vi "Write_ERD_Data_to_File.vi"(0 "refnum in":refnum<file>, 7 "ERD_Data_Bundled_In":T1, 11 "Error In":errorcluster) -> (4 "refnum out":refnum<file>, 15 "Error Out":errorcluster)   [LabVIEW 2014]
uses:
  type defs/ERD_Data_Bundled.ctl
  type defs/ATC_Data.ctl
  type defs/Redundant.ctl
  type defs/Version.ctl
  type defs/Algorithms.ctl
  type defs/ERD_Always_Show.ctl
  type defs/Fault_Table_Info.ctl
  type defs/Cycle_Diag.ctl
panel:
  # "Wet Load Size"
  # "Dry Load Size"
  # "OOB"
  # "Software Version"
  # "Critical Version"
  # "Non-Critical"
  # "XML Crit Ver"
  # "XML Non-Crit"
  # "Daily Build"
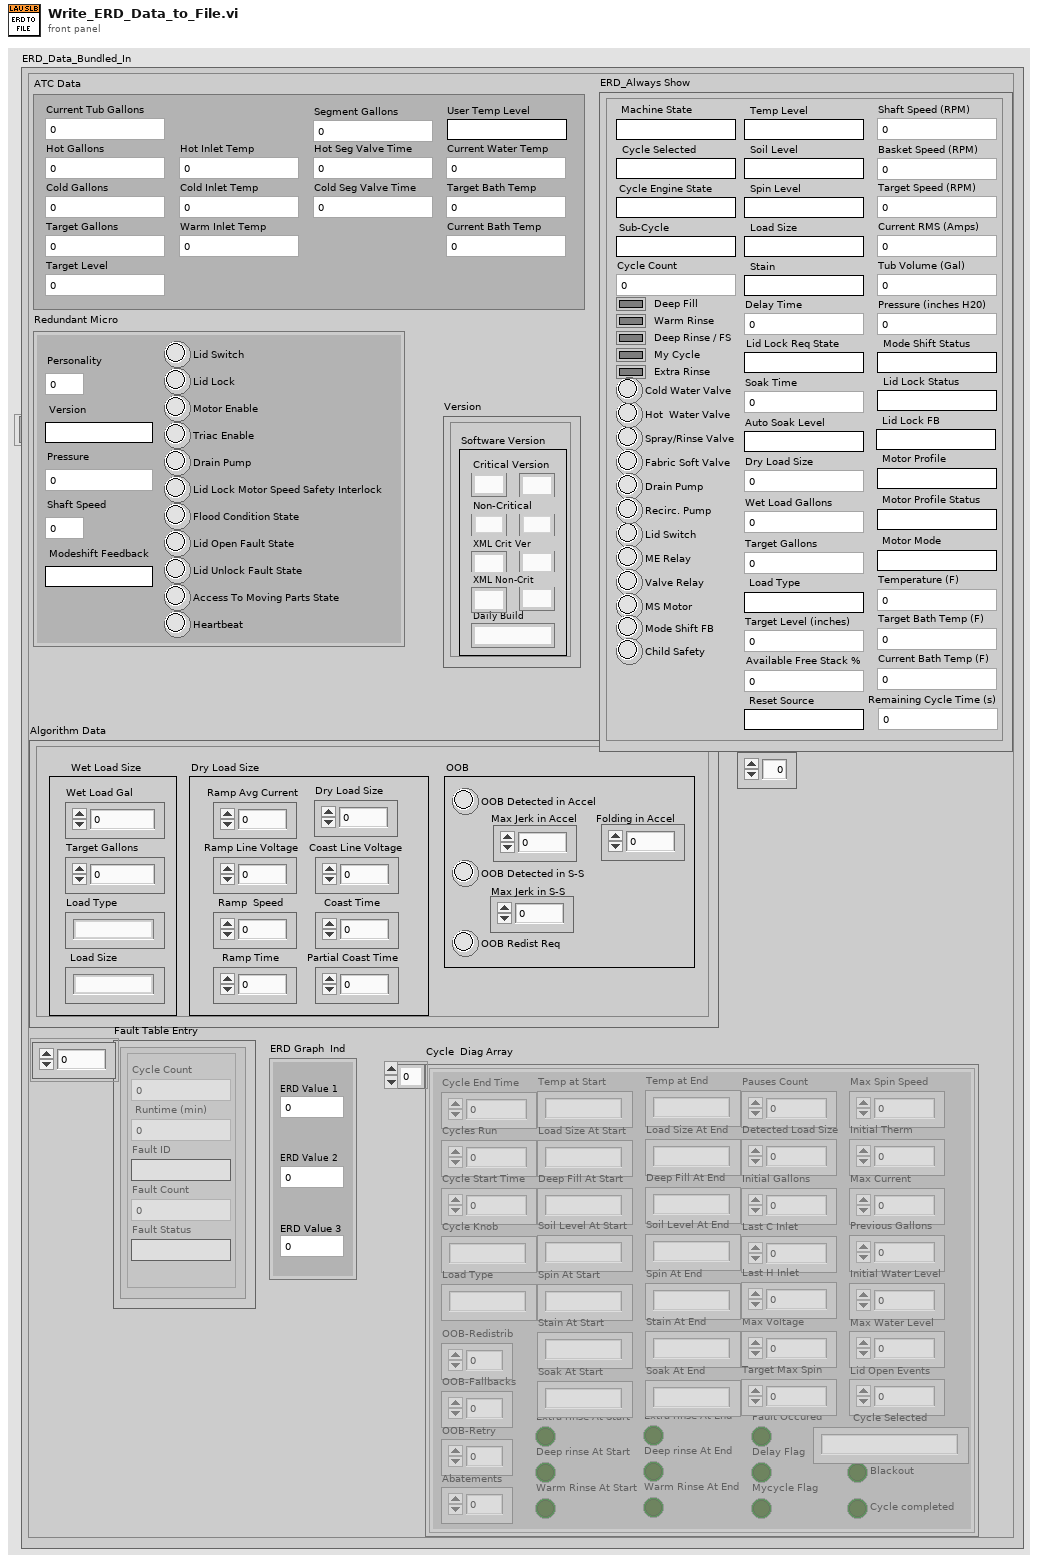
[diagram p1: front panel]
types:
  T1 = typedef "ERD_Data_Bundled.ctl" = cluster{"ATC Data":T2, "Redundant Micro":T3, "Version":T4, "Algorithm Data":T5, "ERD_Always Show":T6, "ERD Graph  Ind":cluster{"ERD Value 1":dbl, "ERD Value 2":dbl, "ERD Value 3":dbl}, "Personality Set":u8, "Fault Table Entry":T7[], "Cycle  Diag Array":T8[]}
  T2 = typedef "ATC_Data.ctl" = cluster{"Current Tub Gallons":dbl, "Hot Gallons":dbl, "Cold Gallons":dbl, "Target Gallons":dbl, "Current Water Temp":dbl, "Target Level":u32, "Target Bath Temp":dbl, "Current Bath Temp ":dbl, "Cold Inlet Temp":dbl, "Hot Inlet Temp":dbl, "Warm Inlet Temp":dbl, "Hot Seg Valve Time":u16, "Cold Seg Valve Time ":u16, "User Temp Level":string, "Segment Gallons":dbl}
  T3 = typedef "Redundant.ctl" = cluster{"Version":string, "Personality":u8, "Pressure ":dbl, "Shaft Speed":u16, "Modeshift Feedback":string, "Lid Switch":bool, "Lid Lock":bool, "Triac Enable":bool, "Drain Pump":bool, "Lid Lock Motor Speed Safety Interlock":bool, "Flood Condition State":bool, "Lid Open Fault State":bool, "Access To Moving Parts State":bool, "Heartbeat":bool, "Motor Enable":bool, "Lid Unlock Fault State":bool}
  T4 = typedef "Version.ctl" = cluster{"Critical Major":string, "Critical Minor":string, "Non-Critical Minor":string, "Non-Critical Major":string, "XML Crit Minor":string, "XMLCrit Major":string, "Daily Rev":string, "XML Non-crit Minor":string, "Xml Non-crit Major":string}
  T5 = typedef "Algorithms.ctl" = cluster{"Wet Load Gal":dbl, "Target Gallons":dbl, "Load Type":string, "Load Size":string, "Coast Time":u16, "Ramp Time":u16, "Ramp  Speed":u16, "Ramp Avg Current":dbl, "OOB Redist Req":bool, "OOB Detected in S-S":bool, "Folding in Accel":i32, "Max Jerk in Accel":i32, "Max Jerk in S-S":i32, "OOB Detected in Accel":bool, "Partial Coast Time":u16, "Dry Load Size":dbl, "Ramp Line Voltage ":dbl, "Coast Line Voltage":dbl}
  T6 = typedef "ERD_Always_Show.ctl" = cluster{"Basket Speed (RPM)":u16, "Machine State":string, "Tub Volume (Gal)":dbl, "Pressure (inches H20)":dbl, "Lid Switch ":bool, "Current RMS (Amps)":dbl, "Cycle Selected":string, "Lid Lock Status":string, "Mode Shift Status":string, "Spray/Rinse Valve":bool, "Fabric Soft Valve":bool, "Drain Pump":bool, "Recirc. Pump":bool, "Cycle Engine State":string, "Hot  Water Valve":bool, "Cold Water Valve":bool, "Motor Profile":string, "Motor Profile Status":string, "Motor Mode":string, "ME Relay":bool, "Cycle Count":u32, "Deep Rinse / FS":bool, "My Cycle":bool, "Soil Level":string, "Spin Level":string, "Stain":string, "Temp Level":string, "Load Size":string, "Delay Time":u16, "Soak Time":u16, "Deep Fill":bool, "Warm Rinse":bool, "Auto Soak Level":string, "Extra Rinse":bool, "Wet Load Gallons":dbl, "Target Gallons":dbl, "Sub-Cycle":string, "Load Type":string, "Target Level (inches)":u32, "Valve Relay":bool, "Dry Load Size":dbl, "Shaft Speed (RPM) ":u16, "MS Motor":bool, "Mode Shift FB":bool, "Target Bath Temp (F)":dbl, "Temperature (F)":dbl, "Current Bath Temp (F)":dbl, "Lid Lock FB":string, "Lid Lock Req State":string, "Remaining Cycle Time (s)":u32, "Available Free Stack %":u8, "Child Safety":bool, "Target Speed (RPM)":u16, "Reset Source":string}
  T7 = typedef "Fault_Table_Info.ctl" = cluster{"Cycle Count":u32, " Runtime (min) ":u32, "Fault Status":string, "Fault ID":string, "Fault Count":u16}
  T8 = typedef "Cycle_Diag.ctl" = cluster{"Cycle End Time":u32, "Cycles Run":u32, "Cycle Start Time":u32, "Cycle Knob":string, "Load Type":string, "OOB-Redistrib":u8, "OOB-Fallbacks":u8, "OOB-Retry":u8, "Temp at Start":string, "Load Size At Start":string, "Deep Fill At Start":string, "Soil Level At Start":string, "Spin At Start":string, "Extra rinse At Start":bool, "Deep rinse At Start":bool, "Stain At Start":string, "Soak At Start":string, "Warm Rinse At Start":bool, "Temp at End":string, "Load Size At End":string, "Deep Fill At End":string, "Soil Level At End":string, "Spin At End":string, "Extra rinse At End":bool, "Deep rinse At End":bool, "Stain At End":string, "Soak At End":string, "Warm Rinse At End":bool, "Pauses Count":u8, "Fault Occured":bool, "Delay Flag":bool, "Mycycle Flag":bool, "Blackout":bool, "Cycle completed":bool, "Detected Load Size":dbl, "Initial Gallons":dbl, "Last C Inlet ":dbl, "Max Voltage":dbl, "Target Max Spin":u16, "Max Spin Speed":u16, "Initial Therm":dbl, "Max Current":dbl, "Previous Gallons":dbl, "Initial Water Level":dbl, "Max Water Level":dbl, "Abatements ":u8, "Lid Open Events":u8, "Cycle Selected":string, "Last H Inlet ":dbl}
  T9 = cluster{"ERD Value 1":dbl, "ERD Value 2":dbl, "ERD Value 3":dbl}
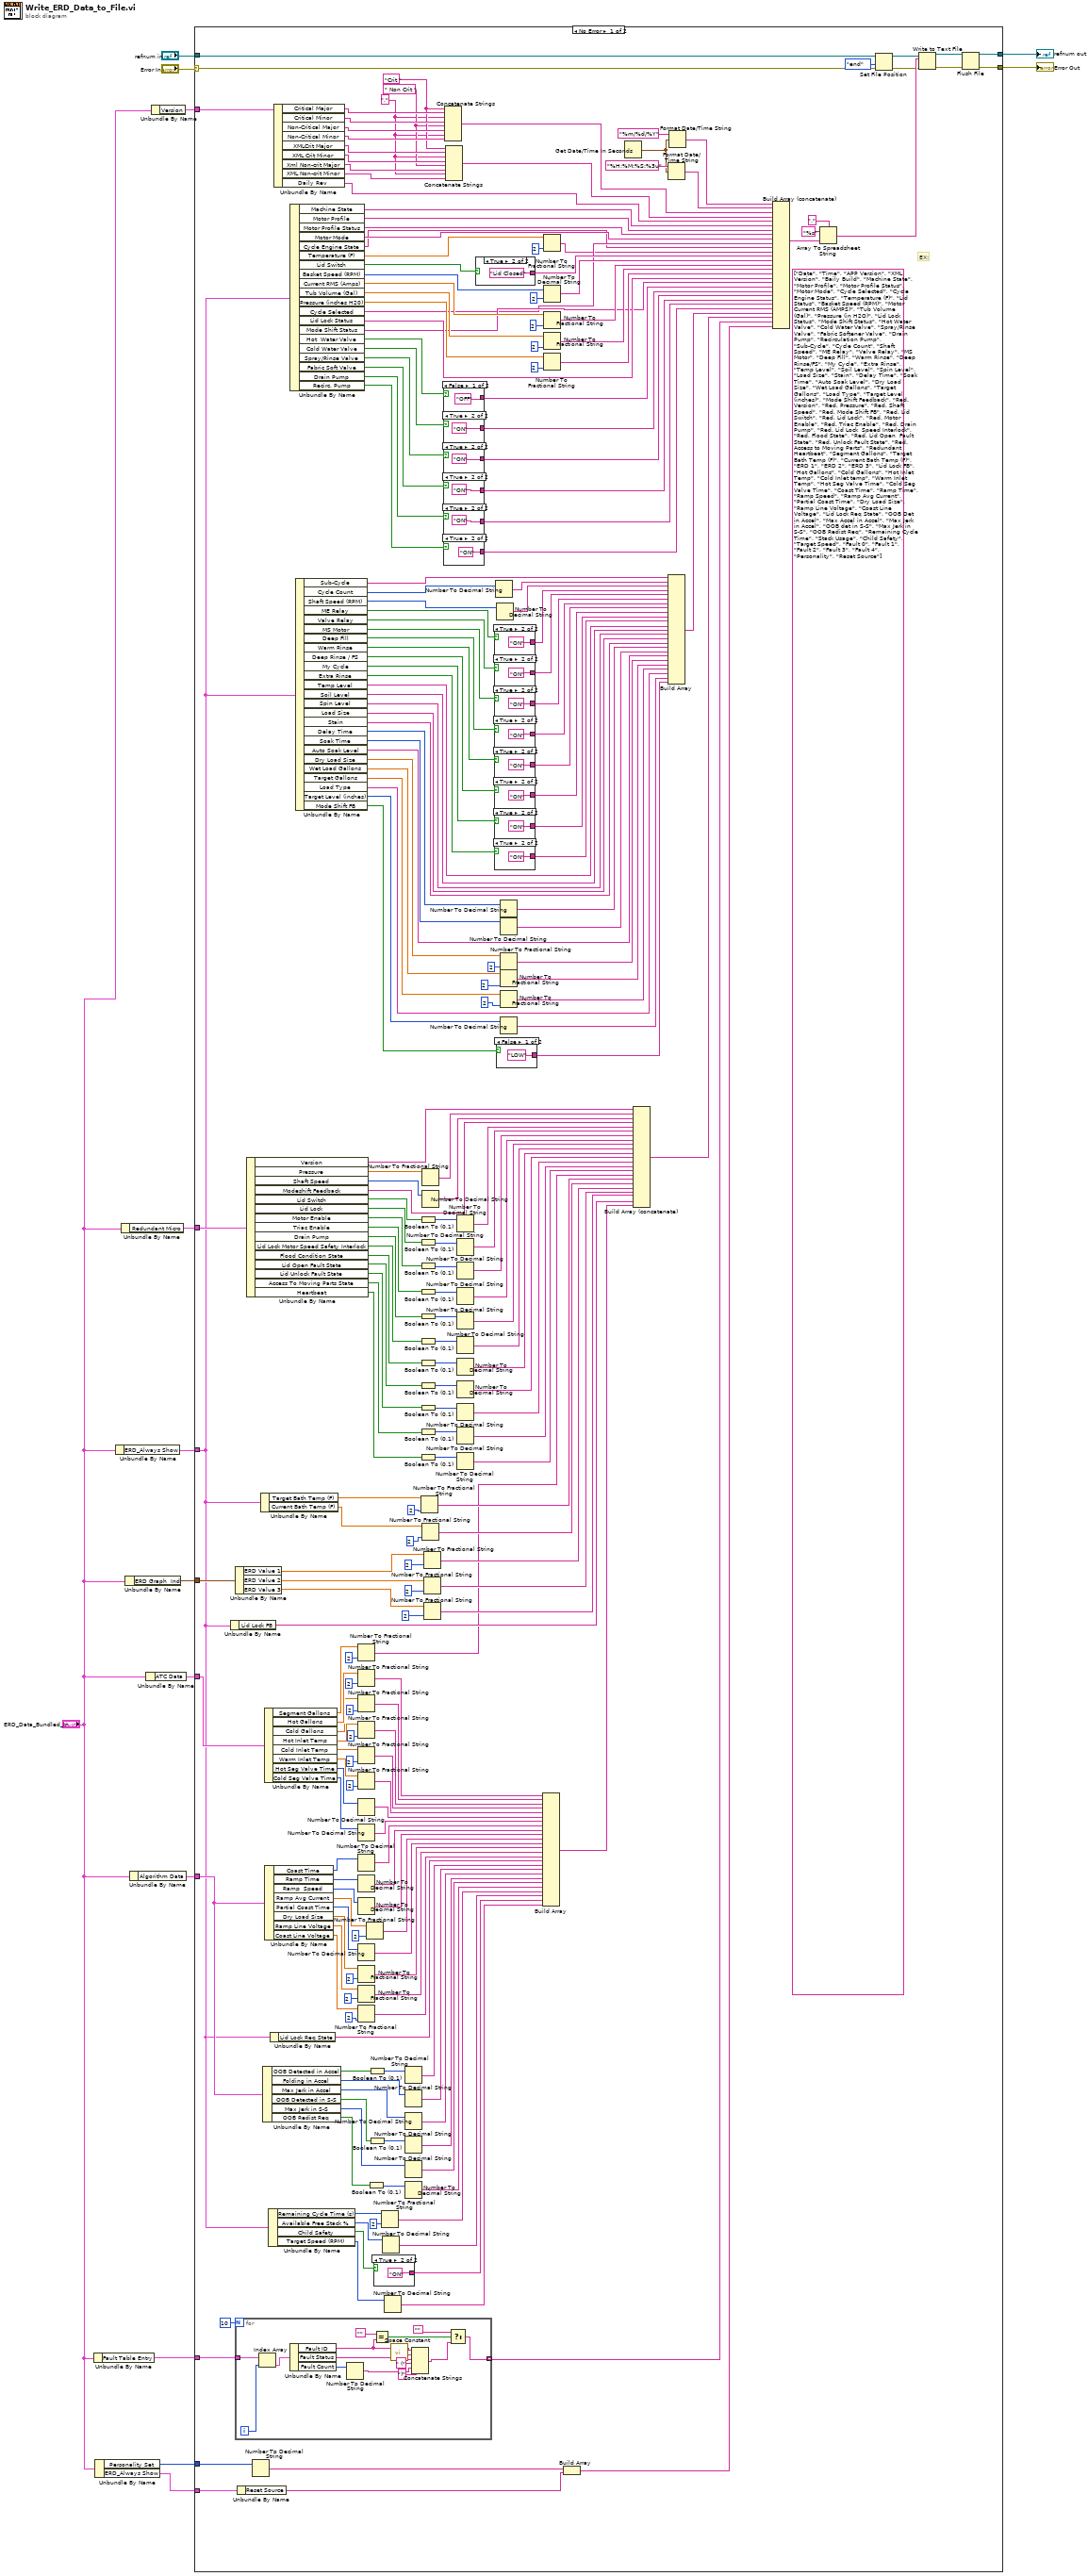
[diagram p0: block diagram]
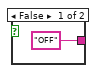
[diagram p2: hidden frame]
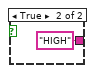
[diagram p3: hidden frame]
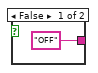
[diagram p4: hidden frame]
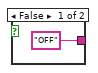
[diagram p5: hidden frame]
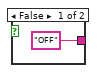
[diagram p6: hidden frame]
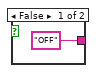
[diagram p7: hidden frame]
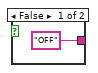
[diagram p8: hidden frame]
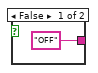
[diagram p9: hidden frame]
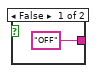
[diagram p10: hidden frame]
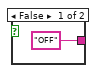
[diagram p11: hidden frame]
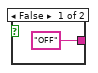
[diagram p12: hidden frame]
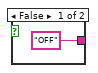
[diagram p13: hidden frame]
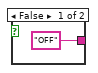
[diagram p14: hidden frame]
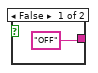
[diagram p15: hidden frame]
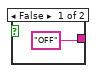
[diagram p16: hidden frame]
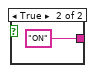
[diagram p17: hidden frame]
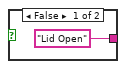
[diagram p18: hidden frame]
diagram:
  n1 = Unbundle By Name("ERD_Data_Bundled_In") -> ("Fault Table Entry"=w1:T7[])
  n2 = Unbundle By Name("ERD_Data_Bundled_In") -> ("Personality Set"=w3:u8, "ERD_Always Show"=w2:T6)
  n3 = Unbundle By Name("ERD_Data_Bundled_In") -> ("ERD_Always Show"=w7:T6)
  n4 = Unbundle By Name("ERD_Data_Bundled_In") -> ("Redundant Micro"=w8:T3)
  n5 = Unbundle By Name("ERD_Data_Bundled_In") -> ("ERD Graph  Ind"=w5:T9)
  n6 = Unbundle By Name("ERD_Data_Bundled_In") -> ("Algorithm Data"=w9:T5)
  n7 = Unbundle By Name("ERD_Data_Bundled_In") -> ("ATC Data"=w10:T2)
  n8 = Unbundle By Name("ERD_Data_Bundled_In") -> ("Version"=w6:T4)
  n9 = case shown="No Error" "Error In" {
    selector: "Error In" -> [w232 w318]
    tunnel: [w24 w317] -> w13
    tunnel: "refnum in" -> [w235 w317]
    tunnel: [w23 w318] -> w11
    tunnel: w6 -> [w174 _]
    tunnel: w8 -> [w157 _]
    tunnel: w5 -> [w112 _]
    tunnel: w10 -> [w104 _]
    tunnel: w9 -> [w71 _]
    tunnel: w7 -> [w22 _]
    tunnel: w3 -> [w21 _]
    tunnel: w2 -> [w20 _]
    tunnel: w1 -> [w16 _]
    frame No Error {
      (unwired) string[] ["Date", "Time", "APP Version", "XML Version", "Baily Build", "Machine State", "Motor Profile", "Motor Profile Status", "Motor Mode", "Cycle Selected", "Cycle Engine Status", "Temperature (F)", "Lid Status", "Basket Speed (RPM)", "Motor Current RMS (AMPS)", "Tub Volume (Gal)", "Pressure (in H2O)", "Lid Lock Status", "Mode Shift Status", "Hot Water Valve", "Cold Water Valve", "Spray/Rinse Valve", "Fabric Softener Valve", "Drain Pump", "Recirculation Pump", "Sub-Cycle", "Cycle Count", "Shaft Speed", "ME Relay", "Valve Relay", "MS Motor", "Deep Fill", "Warm Rinse", "Deep Rinse/FS", "My Cycle", "Extra Rinse", "Temp Level", "Soil Level", "Spin Level", "Load Size", "Stain", "Delay Time", "Soak Time", "Auto Soak Level", "Dry Load Size", "Wet Load Gallons", "Target Gallons", "Load Type", "Target Level (inches)", "Mode Shift Feedback", "Red. Version", "Red. Pressure", "Red. Shaft Speed", "Red. Mode Shift FB", "Red. Lid Switch", "Red. Lid Lock", "Red. Motor Enable", "Red. Triac Enable", "Red. Drain Pump", "Red. Lid Lock  Speed Interlock", "Red. Flood State", "Red. Lid Open  Fault State", "Red. Unlock Fault State", "Red. Access to Moving Parts", "Redundant Heartbeat", "Segment Gallons", "Target Bath Temp (F)", "Current Bath Temp (F)", "ERD 1", "ERD 2", "ERD 3", "Lid Lock FB", "Hot Gallons", "Cold Gallons", "Hot Inlet Temp", "Cold Inlet temp", "Warm Inlet Temp", "Hot Seg Valve Time", "Cold Seg Valve Time", "Coast Time", "Ramp Time", "Ramp Speed", "Ramp Avg Current", "Partial Coast Time", "Dry Load Size", "Ramp Line Voltage", "Coast Line Voltage", "Lid Lock Req State", "OOB Det in Accel", "Max Accel in Accel", "Max Jerk in Accel", "OOB det in S-S", "Max Jerk in S-S", "OOB Redist Req", "Remaining Cycle Time", "Stack Usage", "Child Safety", "Target Speed", "Fault 0", "Fault 1", "Fault 2", "Fault 3", "Fault 4", "Personality", "Reset Source"]
      w166 = " Non Crit " ("element")
      w164 = "." ("element")
      w169 = "Crit " ("element")
      # "EX:"
      n10 = Unbundle By Name(w22) -> ("Lid Lock FB"=w105:string)
      n11 = Unbundle By Name(w112) -> ("ERD Value 1"=w111:dbl, "ERD Value 2"=w110:dbl, "ERD Value 3"=w109:dbl)
      n12 = for {
        N: 10 -> [_]
        tunnel: [w272] -> w27 mode=indexing
        tunnel: w16 -> [w270]
        i -> [w268]
        n13 = Index Array(array=w270, index=w268) -> (element=w269:T7)
        n14 = Unbundle By Name(w269) -> ("Fault ID"=w275:string, "Fault Status"=w280:string, "Fault Count"=w282:u16)
        n15 = Number To Decimal String(number=w282) -> (decimal integer string=w278:string)  [unwired: 1 in]
        n16 = Equal?(x="", y=w275) -> (x = y?=w274:bool)
        n17 = call <vilib>:"Space Constant.vi"() -> ("String"=w281:string)
        n18 = Concatenate Strings(w275, w281, w280, " (" ("string"), w278, ")" ("string")) -> (w273:string)
        n19 = Select(t="", s=w274, f=w273) -> (s? t:f=w272:string)
      }
      n20 = Unbundle By Name(w20) -> ("Reset Source"=w18:string)
      n21 = Unbundle By Name(w157) -> ("Version"=w156:string, "Pressure"=w155:dbl, "Shaft Speed"=w153:u16, "Modeshift Feedback"=w151:string, "Lid Switch"=w148:bool, "Lid Lock"=w138:bool, "Motor Enable"=w137:bool, "Triac Enable"=w136:bool, "Drain Pump"=w135:bool, "Lid Lock Motor Speed Safety Interlock"=w134:bool, "Flood Condition State"=w133:bool, "Lid Open Fault State"=w132:bool, "Lid Unlock Fault State"=w130:bool, "Access To Moving Parts State"=w129:bool, "Heartbeat"=w128:bool)
      n22 = Number To Decimal String(number=w21) -> (decimal integer string=w19:string)  [unwired: 1 in]
      n23 = Unbundle By Name(w22) -> ("Target Bath Temp (F)"=w116:dbl, "Current Bath Temp (F)"=w114:dbl)
      n24 = Unbundle By Name(w71) -> ("OOB Detected in Accel"=w69:bool, "Folding in Accel"=w67:i32, "Max Jerk in Accel"=w65:i32, "OOB Detected in S-S"=w63:bool, "Max Jerk in S-S"=w62:i32, "OOB Redist Req"=w60:bool)
      n25 = Unbundle By Name(w104) -> ("Segment Gallons"=w38:dbl, "Hot Gallons"=w103:dbl, "Cold Gallons"=w102:dbl, "Hot Inlet Temp"=w101:dbl, "Cold Inlet Temp"=w100:dbl, "Warm Inlet Temp"=w99:dbl, "Hot Seg Valve Time"=w98:u16, "Cold Seg Valve Time"=w97:u16)
      n26 = Unbundle By Name(w71) -> ("Coast Time"=w88:u16, "Ramp Time"=w87:u16, "Ramp  Speed"=w86:u16, "Ramp Avg Current"=w85:dbl, "Partial Coast Time"=w84:u16, "Dry Load Size"=w83:dbl, "Ramp Line Voltage"=w82:dbl, "Coast Line Voltage"=w81:dbl)
      n27 = Unbundle By Name(w22) -> ("Remaining Cycle Time (s)"=w35:u32, "Available Free Stack %"=w33:u8, "Child Safety"=w31:bool, "Target Speed (RPM)"=w29:u16)
      n28 = Unbundle By Name(w22) -> ("Lid Lock Req State"=w72:string)
      n29 = Unbundle By Name(w174) -> ("Critical Major"=w173:string, "Critical Minor"=w172:string, "Non-Critical Major"=w171:string, "Non-Critical Minor"=w170:string, "XMLCrit Major"=w168:string, "XML Crit Minor"=w167:string, "Xml Non-crit Major"=w165:string, "XML Non-crit Minor"=w163:string, "Daily Rev"=w158:string)
      n30 = Unbundle By Name(w22) -> ("Machine State"=w266:string, "Motor Profile"=w265:string, "Motor Profile Status"=w226:string, "Motor Mode"=w224:string, "Cycle Engine State"=w220:string, "Temperature (F)"=w225:dbl, "Lid Switch"=w257:bool, "Basket Speed (RPM)"=w258:u16, "Current RMS (Amps)"=w250:dbl, "Tub Volume (Gal)"=w261:dbl, "Pressure (inches H20)"=w260:dbl, "Cycle Selected"=w221:string, "Lid Lock Status"=w249:string, "Mode Shift Status"=w248:string, "Hot  Water Valve"=w247:bool, "Cold Water Valve"=w246:bool, "Spray/Rinse Valve"=w245:bool, "Fabric Soft Valve"=w244:bool, "Drain Pump"=w239:bool, "Recirc. Pump"=w238:bool)
      n31 = Unbundle By Name(w22) -> ("Sub-Cycle"=w218:string, "Cycle Count"=w217:u32, "Shaft Speed (RPM)"=w215:u16, "ME Relay"=w213:bool, "Valve Relay"=w212:bool, "MS Motor"=w211:bool, "Deep Fill"=w210:bool, "Warm Rinse"=w209:bool, "Deep Rinse / FS"=w208:bool, "My Cycle"=w207:bool, "Extra Rinse"=w206:bool, "Temp Level"=w198:string, "Soil Level"=w197:string, "Spin Level"=w196:string, "Load Size"=w195:string, "Stain"=w194:string, "Delay Time"=w193:u16, "Soak Time"=w192:u16, "Auto Soak Level"=w191:string, "Dry Load Size"=w190:dbl, "Wet Load Gallons"=w189:dbl, "Target Gallons"=w188:dbl, "Load Type"=w182:string, "Target Level (inches)"=w180:u32, "Mode Shift FB"=w178:bool)
      n32 = Number To Fractional String(number=w38, precision (6)=i16 2) -> (F-format string=w37:string)  [unwired: 2 in]
      n33 = Number To Fractional String(number=w103, precision (6)=i16 2) -> (F-format string=w96:string)  [unwired: 2 in]
      n34 = Number To Fractional String(number=w102, precision (6)=i16 2) -> (F-format string=w95:string)  [unwired: 2 in]
      n35 = Number To Fractional String(number=w101, precision (6)=i16 2) -> (F-format string=w94:string)  [unwired: 2 in]
      n36 = Number To Fractional String(number=w100, precision (6)=i16 2) -> (F-format string=w93:string)  [unwired: 2 in]
      n37 = Number To Fractional String(number=w99, precision (6)=i16 2) -> (F-format string=w92:string)  [unwired: 2 in]
      n38 = Number To Decimal String(number=w98) -> (decimal integer string=w91:string)  [unwired: 1 in]
      n39 = Number To Decimal String(number=w97) -> (decimal integer string=w90:string)  [unwired: 1 in]
      n40 = Number To Decimal String(number=w88) -> (decimal integer string=w80:string)  [unwired: 1 in]
      n41 = Number To Decimal String(number=w87) -> (decimal integer string=w79:string)  [unwired: 1 in]
      n42 = Number To Decimal String(number=w86) -> (decimal integer string=w78:string)  [unwired: 1 in]
      n43 = Number To Decimal String(number=w84) -> (decimal integer string=w76:string)  [unwired: 1 in]
      n44 = Number To Fractional String(number=w83, precision (6)=i16 2) -> (F-format string=w75:string)  [unwired: 2 in]
      n45 = Number To Fractional String(number=w82, precision (6)=i16 2) -> (F-format string=w74:string)  [unwired: 2 in]
      n46 = Number To Fractional String(number=w81, precision (6)=i16 2) -> (F-format string=w73:string)  [unwired: 2 in]
      n47 = Number To Fractional String(number=w85, precision (6)=i16 2) -> (F-format string=w77:string)  [unwired: 2 in]
      n48 = Boolean To (0,1)(Boolean=w60) -> (0, 1=w61:i16)
      n49 = Boolean To (0,1)(Boolean=w69) -> (0, 1=w70:i16)
      n50 = Boolean To (0,1)(Boolean=w63) -> (0, 1=w64:i16)
      n51 = case shown="True" w31 {
        tunnel: ["OFF" "ON"] -> w30
        frame False {
        }
        frame True {
        }
      }
      n52 = Number To Fractional String(number=w35, precision (6)=i16 2) -> (F-format string=w34:string)  [unwired: 2 in]
      n53 = Number To Decimal String(number=w33) -> (decimal integer string=w32:string)  [unwired: 1 in]
      n54 = Number To Decimal String(number=w29) -> (decimal integer string=w28:string)  [unwired: 1 in]
      n55 = Number To Decimal String(number=w70) -> (decimal integer string=w68:string)  [unwired: 1 in]
      n56 = Number To Decimal String(number=w67) -> (decimal integer string=w66:string)  [unwired: 1 in]
      n57 = Number To Decimal String(number=w65) -> (decimal integer string=w59:string)  [unwired: 1 in]
      n58 = Number To Decimal String(number=w64) -> (decimal integer string=w58:string)  [unwired: 1 in]
      n59 = Number To Decimal String(number=w62) -> (decimal integer string=w57:string)  [unwired: 1 in]
      n60 = Number To Decimal String(number=w61) -> (decimal integer string=w56:string)  [unwired: 1 in]
      n61 = Boolean To (0,1)(Boolean=w148) -> (0, 1=w150:i16)
      n62 = Boolean To (0,1)(Boolean=w138) -> (0, 1=w147:i16)
      n63 = Boolean To (0,1)(Boolean=w137) -> (0, 1=w146:i16)
      n64 = Boolean To (0,1)(Boolean=w136) -> (0, 1=w145:i16)
      n65 = Boolean To (0,1)(Boolean=w135) -> (0, 1=w144:i16)
      n66 = Boolean To (0,1)(Boolean=w134) -> (0, 1=w143:i16)
      n67 = Boolean To (0,1)(Boolean=w133) -> (0, 1=w142:i16)
      n68 = Boolean To (0,1)(Boolean=w132) -> (0, 1=w141:i16)
      n69 = Boolean To (0,1)(Boolean=w130) -> (0, 1=w140:i16)
      n70 = Boolean To (0,1)(Boolean=w129) -> (0, 1=w139:i16)
      n71 = Boolean To (0,1)(Boolean=w128) -> (0, 1=w131:i16)
      n72 = Number To Fractional String(number=w116, precision (6)=i16 2) -> (F-format string=w115:string)  [unwired: 2 in]
      n73 = Number To Fractional String(number=w114, precision (6)=i16 2) -> (F-format string=w113:string)  [unwired: 2 in]
      n74 = Number To Fractional String(number=w155) -> (F-format string=w154:string)  [unwired: 3 in]
      n75 = Number To Decimal String(number=w153) -> (decimal integer string=w152:string)  [unwired: 1 in]
      n76 = Number To Fractional String(number=w111, precision (6)=i16 2) -> (F-format string=w108:string)  [unwired: 2 in]
      n77 = Number To Fractional String(number=w110, precision (6)=i16 2) -> (F-format string=w107:string)  [unwired: 2 in]
      n78 = Number To Fractional String(number=w109, precision (6)=i16 2) -> (F-format string=w106:string)  [unwired: 2 in]
      n79 = case shown="False" w247 {
        tunnel: ["OFF" "ON"] -> w243
        frame False {
        }
        frame True {
        }
      }
      n80 = case shown="True" w246 {
        tunnel: ["OFF" "ON"] -> w222
        frame False {
        }
        frame True {
        }
      }
      n81 = case shown="True" w245 {
        tunnel: ["OFF" "ON"] -> w242
        frame False {
        }
        frame True {
        }
      }
      n82 = case shown="True" w244 {
        tunnel: ["OFF" "ON"] -> w241
        frame False {
        }
        frame True {
        }
      }
      n83 = case shown="True" w239 {
        tunnel: ["OFF" "ON"] -> w240
        frame False {
        }
        frame True {
        }
      }
      n84 = case shown="True" w238 {
        tunnel: ["OFF" "ON"] -> w223
        frame False {
        }
        frame True {
        }
      }
      n85 = Concatenate Strings(w169, w173, w164, w172, w166, w171, w164, w170) -> (w160:string)
      n86 = Concatenate Strings(w169, w168, w164, w167, w166, w165, w164, w163) -> (w159:string)
      n87 = Number To Decimal String(number=w150) -> (decimal integer string=w149:string)  [unwired: 1 in]
      n88 = Number To Decimal String(number=w147) -> (decimal integer string=w127:string)  [unwired: 1 in]
      n89 = Number To Decimal String(number=w146) -> (decimal integer string=w126:string)  [unwired: 1 in]
      n90 = Number To Decimal String(number=w145) -> (decimal integer string=w125:string)  [unwired: 1 in]
      n91 = Number To Decimal String(number=w144) -> (decimal integer string=w124:string)  [unwired: 1 in]
      n92 = Number To Decimal String(number=w143) -> (decimal integer string=w123:string)  [unwired: 1 in]
      n93 = Number To Decimal String(number=w142) -> (decimal integer string=w122:string)  [unwired: 1 in]
      n94 = Number To Decimal String(number=w141) -> (decimal integer string=w121:string)  [unwired: 1 in]
      n95 = Number To Decimal String(number=w140) -> (decimal integer string=w120:string)  [unwired: 1 in]
      n96 = Number To Decimal String(number=w139) -> (decimal integer string=w119:string)  [unwired: 1 in]
      n97 = Number To Decimal String(number=w131) -> (decimal integer string=w118:string)  [unwired: 1 in]
      n98 = case shown="True" w257 {
        tunnel: ["Lid Open" "Lid Closed"] -> w256
        frame False {
        }
        frame True {
        }
      }
      n99 = case shown="True" w213 {
        tunnel: ["OFF" "ON"] -> w205
        frame False {
        }
        frame True {
        }
      }
      n100 = case shown="True" w212 {
        tunnel: ["OFF" "ON"] -> w204
        frame False {
        }
        frame True {
        }
      }
      n101 = case shown="True" w211 {
        tunnel: ["OFF" "ON"] -> w203
        frame False {
        }
        frame True {
        }
      }
      n102 = case shown="True" w210 {
        tunnel: ["OFF" "ON"] -> w202
        frame False {
        }
        frame True {
        }
      }
      n103 = case shown="True" w209 {
        tunnel: ["OFF" "ON"] -> w201
        frame False {
        }
        frame True {
        }
      }
      n104 = case shown="True" w208 {
        tunnel: ["OFF" "ON"] -> w200
        frame False {
        }
        frame True {
        }
      }
      n105 = case shown="True" w207 {
        tunnel: ["OFF" "ON"] -> w199
        frame False {
        }
        frame True {
        }
      }
      n106 = case shown="True" w206 {
        tunnel: ["OFF" "ON"] -> w176
        frame False {
        }
        frame True {
        }
      }
      n107 = Number To Decimal String(number=w217) -> (decimal integer string=w216:string)  [unwired: 1 in]
      n108 = Number To Decimal String(number=w215) -> (decimal integer string=w214:string)  [unwired: 1 in]
      n109 = case shown="False" w178 {
        tunnel: ["LOW" "HIGH"] -> w177
        frame False {
        }
        frame True {
        }
      }
      n110 = Number To Decimal String(number=w193) -> (decimal integer string=w187:string)  [unwired: 1 in]
      n111 = Number To Decimal String(number=w192) -> (decimal integer string=w186:string)  [unwired: 1 in]
      n112 = Number To Fractional String(number=w190, precision (6)=i16 2) -> (F-format string=w185:string)  [unwired: 2 in]
      n113 = Number To Fractional String(number=w189, precision (6)=i16 2) -> (F-format string=w184:string)  [unwired: 2 in]
      n114 = Number To Fractional String(number=w188, precision (6)=i16 2) -> (F-format string=w183:string)  [unwired: 2 in]
      n115 = Number To Decimal String(number=w180) -> (decimal integer string=w181:string)  [unwired: 1 in]
      n116 = Build Array(w96, w95, w94, w93, w92, w91, w90, w80, w79, w78, w77, w76, w75, w74, w73, w72, w68, w66, w59, w58, w57, w56, w34, w32, w30, w28) -> (w89:string[])
      n117 = Number To Fractional String(number=w225, precision (6)=i16 2) -> (F-format string=w219:string)  [unwired: 2 in]
      n118 = Number To Decimal String(number=w258, width (-)=i16 2 ("precision (6)")) -> (decimal integer string=w255:string)
      n119 = Number To Fractional String(number=w250, precision (6)=i16 2) -> (F-format string=w254:string)  [unwired: 2 in]
      n120 = Number To Fractional String(number=w261, precision (6)=i16 2) -> (F-format string=w253:string)  [unwired: 2 in]
      n121 = Number To Fractional String(number=w260, precision (6)=i16 2) -> (F-format string=w252:string)  [unwired: 2 in]
      n122 = Build Array(w19, w18) -> (w17:string[])
      n123 = Get Date/Time In Seconds() -> (seconds since 1Jan1904=w228:timestamp)
      n124 = Build Array (concatenate)(w156, w154, w152, w151, w149, w127, w126, w125, w124, w123, w122, w121, w120, w119, w118, w37, w115, w113, w108, w107, w106, w105, w89) -> (w117:string[])
      n125 = Format Date/Time String(time format string (%c)="%H:%M:%S:%3u", seconds (now)=w228) -> (date/time string=w161:string)  [unwired: 1 in]
      n126 = Build Array(w218, w216, w214, w205, w204, w203, w202, w201, w200, w199, w176, w198, w197, w196, w195, w194, w187, w186, w191, w185, w184, w183, w182, w181, w177) -> (w179:string[])
      n127 = Format Date/Time String(time format string (%c)="%m/%d/%Y", seconds (now)=w228) -> (date/time string=w162:string)  [unwired: 1 in]
      n128 = Build Array (concatenate)(w162, w161, w160, w159, w158, w266, w265, w226, w224, w221, w220, w219, w256, w255, w254, w253, w252, w249, w248, w243, w222, w242, w241, w240, w223, w179, w117, w27, w17) -> (w227:string[])
      n129 = Array To Spreadsheet String(delimiter (Tab)=",", array=w227, 3:"%s" ("format string")) -> (spreadsheet string=w237:string)
      n130 = Set File Position(refnum=w235, from (0:start)=enum16{"start", "end", "current"}."end", error in=w232) -> (refnum out=w234:refnum<file>, error out=w233:errorcluster)  [unwired: 1 in]
      n131 = Write to Text File(file (use dialog)=w234, text=w237, error in=w233) -> (refnum out=w26:refnum<file>, error out=w25:errorcluster)  [unwired: 1 in, 1 out]
      n132 = Flush File(refnum=w26, error in=w25) -> (refnum out=w24:refnum<file>, error out=w23:errorcluster)
    }
    frame Error {
    }
  }
  "Error Out" <- w11
  "refnum out" <- w13
